vi "Queue.Dequeue.vi"(8 "error in (no error)":errorcluster, 11 "queueName":string) -> (0 "error out":errorcluster, 2 "message":string, 3 "data":variant)   [LabVIEW 2019]
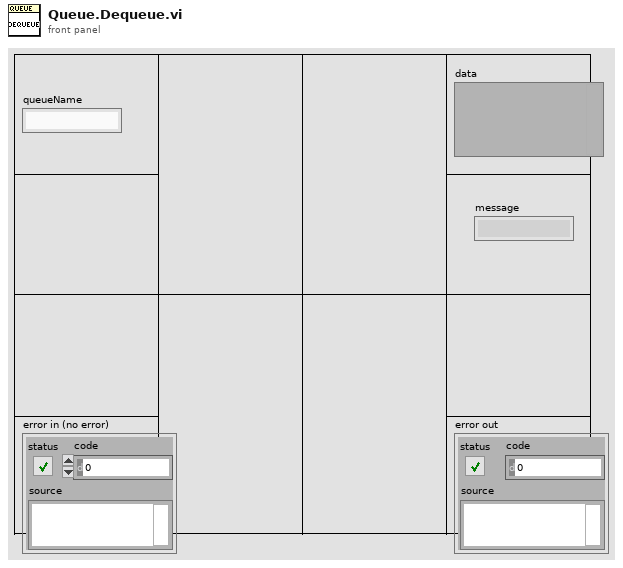
[diagram p1: front panel]
types:
  T1 = typedef "QueueMessage.ctl" = cluster{"message":string, "data":variant}
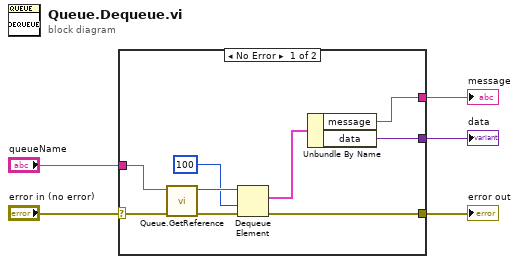
[diagram p0: block diagram]
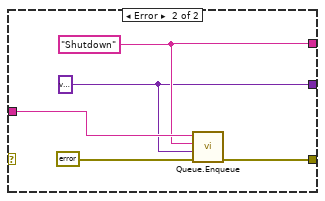
[diagram p2: hidden frame]
diagram:
  n1 = case shown="No Error" "error in (no error)" {
    selector: "error in (no error)" -> [w14 _]
    tunnel: [w12 w17] -> w1
    tunnel: [w8 w16] -> w3
    tunnel: "queueName" -> [w9 w19]
    tunnel: [w7 w15] -> w5
    frame No Error {
      n2 = call "Queue.GetReference.vi"("error in (no error)"=w14, "queueName"=w9) -> ("error out"=w13:errorcluster, "refToQueue"=w11:refnum<queue>)  [unwired: 8 in]
      n3 = Dequeue Element(queue=w11, timeout in ms (-1)=100, error in (no error)=w13) -> (element=w10:T1, error out=w12:errorcluster)  [unwired: 2 out]
      n4 = Unbundle By Name(w10) -> ("message"=w8:string, "data"=w7:variant)
    }
    frame Error {
      w15 = variant
      w16 = "Shutdown"
      n5 = call "Queue.Enqueue.vi"("error in (no error)"=errorcluster {"status"=FALSE, "code"=0, "source"=""}, "data"=w15, "message"=w16, "queueName"=w19) -> ("error out"=w17:errorcluster)  [unwired: 7 in]
    }
  }
  "data" <- w5
  "message" <- w3
  "error out" <- w1
